vi "train_WGAN_D.vi"() -> ()   [LabVIEW 2016]
uses:
  Users/jg754/Documents/Visual Studio 2015/Projects/CLearn/x64/Release/CLearn.dll
panel:
  in  "Real_fake":bool
  in  "last_layer":u32
  in  "first_layer":u32
  in  "gamma":sgl
  in  "adam":bool
  in  "weight_normalization":bool
  in  "batch_update":u32
  in  "lambda":sgl
  out "logits":sgl[][](array[numeric])
  in  "eta":sgl
  in  "buffer array for output":sgl[][](array[numeric])
  in  "input":sgl[][](array[numeric])
  out "ptr out":i64
  out "error":sgl
  in  "ptr":i64
  out "error out":errorcluster
  in  "error in (no error)":errorcluster
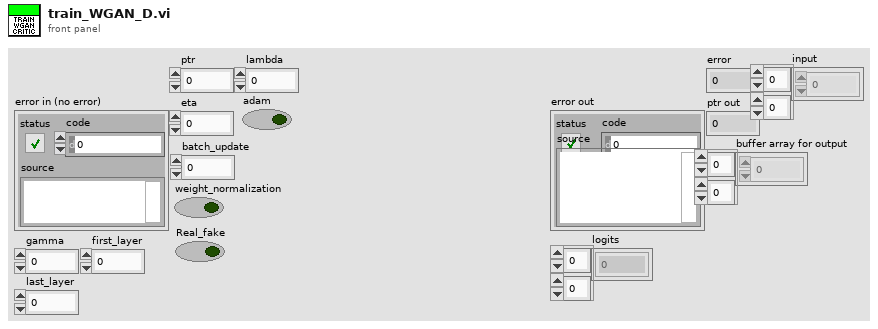
[diagram p1: front panel]
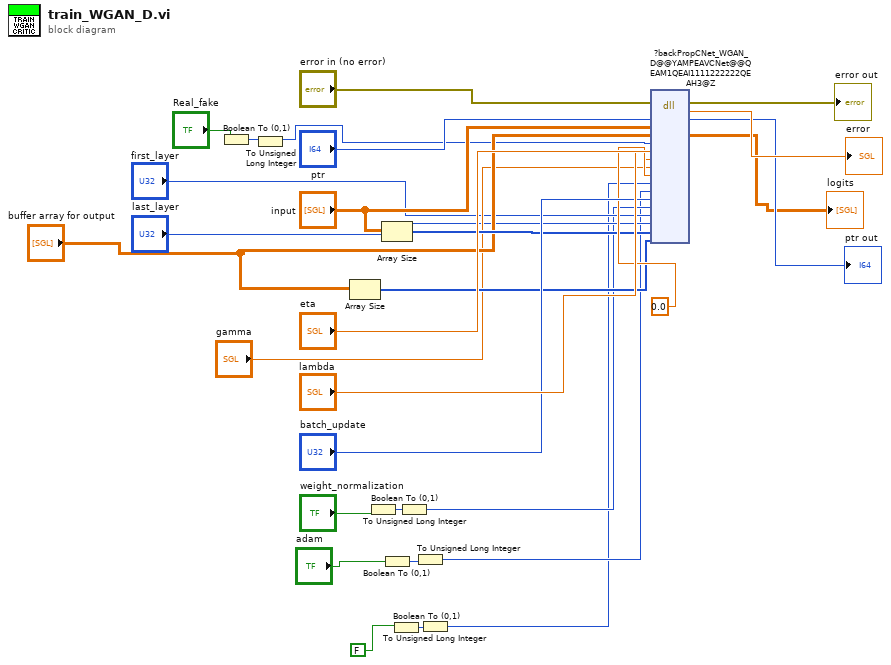
[diagram p0: block diagram]
diagram:
  n1 = Boolean To (0,1)(Boolean="Real_fake") -> (0, 1=w9:i16)
  n2 = To Unsigned Long Integer(number=w9) -> (unsigned 32bit integer=w8:u32)
  n3 = Array Size(array="buffer array for output") -> (size(s)=w14:i32[])
  n4 = Boolean To (0,1)(Boolean="weight_normalization") -> (0, 1=w7:i16)
  n5 = Array Size(array="input") -> (size(s)=w16:i32[])
  n6 = Boolean To (0,1)(Boolean="adam") -> (0, 1=w5:i16)
  n7 = Boolean To (0,1)(Boolean=FALSE) -> (0, 1=w3:i16)
  n8 = To Unsigned Long Integer(number=w7) -> (unsigned 32bit integer=w6:u32)
  n9 = To Unsigned Long Integer(number=w5) -> (unsigned 32bit integer=w4:u32)
  n10 = To Unsigned Long Integer(number=w3) -> (unsigned 32bit integer=w2:u32)
  n11 = dll-call lib="C:/Users/jg754/Documents/Visual Studio 2015/Projects/CLearn/x64/Release/CLearn.dll" fn="?backPropCNet_WGAN_D@@YAMPEAVCNet@@QEAM1QEAI1111222222QEAH3@Z"(error in="error in (no error)", "ptr"="ptr", "input"="input", "outputDesired"="buffer array for output", "real"=w8, "eta"="eta", "metaEta"=sgl 0.0, "gamma"="gamma", "lambda"="lambda", "conjugate"=w2, "adam"=w4, "batch_update"="batch_update", "weight_normalization"=w6, "first_layer"="first_layer", "last_layer"="last_layer", "inFormat"=w16, "outFormat"=w14) -> (error out=→"error out":errorcluster, "error"=→"error":sgl, "ptr"=→"ptr out":i64, "outputDesired"=→"logits":sgl[][])  [unwired: 16 in, 1 out]
